vi "Run PPL Class Load Test.vi"(7 "Show UI on Class load?(T)":bool=TRUE, 8 "error in":errorcluster, 10 "PPL Class Test Plugins":refnum<class "PPL Class Test Plugin.lvclass">[](array[class]), 11 "PPL Name in PPL folder (entire PPL folder if empty)":string) -> (0 "error out":errorcluster, 1 "Success?":bool, 2 "Load Failure":string[](array[string]), 3 "Load Success":string[](array[string]))   [LabVIEW 2020, in "ProjectBuilder.lvlib"]
doc: "Get PPL paths and load the PPLs and see if load succeeds."
uses:
  ProjectBuilder.lvlib
  PPL/HDH.ClassLoader.lvlibp
  PPL Class Test Plugin/PPL Class Test Plugin.lvclass
panel:
  in  "Abort":bool
  out "Current class":string
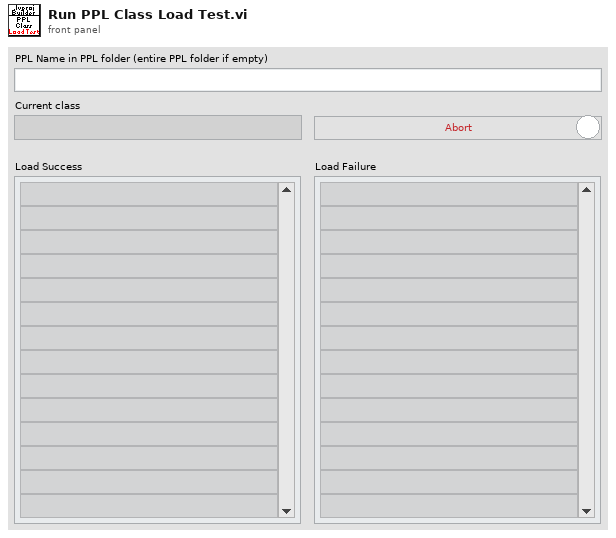
[diagram p1: front panel]
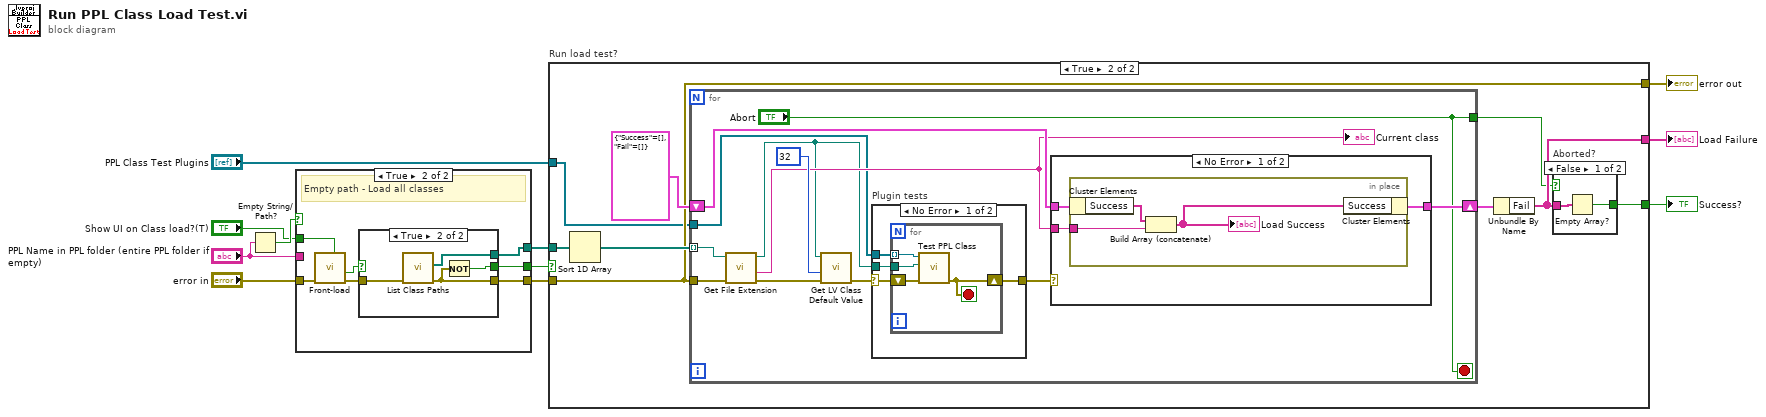
[diagram p0: block diagram]
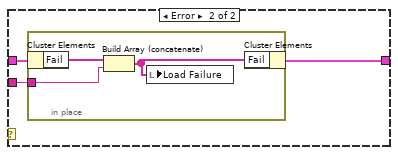
[diagram p5: hidden frame]
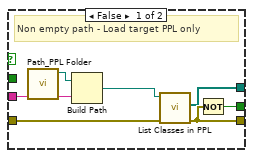
[diagram p6: hidden frame]
diagram:
  n1 = Empty String/Path?(string/path="PPL Name in PPL folder (entire PPL folder if empty)") -> (empty?=w11:bool)
  n2 = case shown="True" w11 {
    tunnel: [w17 w23] -> w8
    tunnel: "error in" -> [w18 w22]
    tunnel: [w16 w21] -> w6
    tunnel: [w15 w20] -> w7
    tunnel: "PPL Name in PPL folder (entire PPL folder if empty)" -> [w13 _]
    tunnel: "Show UI on Class load?(T)" -> [_ w19]
    frame False {
      # "Non empty path - Load target PPL only"
      n3 = call "Path_PPL Folder.vi"() -> ("Data Folder Path"=w14:path)  [unwired: 10 in, 1 out]
      n4 = Build Path(base path=w14, name or relative path=w13) -> (appended path=w12:path)
      n5 = call "List Classes in PPL.vi"("error in"=w18, "PPL Path"=w12) -> ("error out"=w16:errorcluster, "Class Path Array"=w15:path[])  [unwired: 7 in, 1 out]
      n6 = Not(x=w16) -> (.not. x?=w17:bool)
    }
    frame True {
      # "Empty path - Load all classes"
      n7 = call "Front-load.vi"("Show UI?(F)"=w19, "error in (no error)"=w22) -> ("error out"=w25:errorcluster, "Success?"=w24:bool)  [unwired: 8 in]
      n8 = case shown="True" w24 {
        selector: w24 -> [w27 _]
        tunnel: w25 -> [w26 w31]
        tunnel: [w27 w30] -> w23
        tunnel: [w26 w29] -> w21
        tunnel: [_ w28] -> w20
        frame False {
        }
        frame True {
          n9 = call "List Class Paths.vi"("error in (no error)"=w31) -> ("error out"=w29:errorcluster, "Class Paths"=w28:path[])  [unwired: 8 in, 1 out]
          n10 = Not(x=w29) -> (.not. x?=w30:bool)
        }
      }
    }
  }
  n11 = case "Run load test?" shown="True" w8 {
    selector: w8 -> [w33 _]
    tunnel: w7 -> [_ w42]
    tunnel: w6 -> [w32 w36]
    tunnel: [w33 w37] -> w4
    tunnel: [_ w38] -> w5
    tunnel: [w32 w36] -> w3
    tunnel: "PPL Class Test Plugins" -> [_ w34]
    frame False {
    }
    frame True {
      n12 = Sort 1D Array(array=w42) -> (sorted array=w41:path[])
      n13 = for {
        tunnel: w41 -> [w53] mode=indexing
        tunnel: w36 -> [w55]
        shift-right: [w50] -> w40
        shift-left: cluster{"Success":string[], "Fail":string[]} {"Success"=[], "Fail"=[]} -> [w52]
        tunnel: ["Abort"] -> w35
        tunnel: w34 -> [w48]
        stop <- "Abort" stop-if-true
        n14 = call <vilib>:"Get File Extension.vi"("error in (no error)"=w55, "file"=w53) -> ("error out"=w54:errorcluster, "filename without extension"=w51:string, "dup file"=w45:path)  [unwired: 5 in, 2 out]
        "Current class" <- w51
        n15 = call <vilib>:"Get LV Class Default Value.vi"("error in (no error)"=w54, "options"=u32 32, "class path"=w45) -> ("error out"=w47:errorcluster)  [unwired: 7 in, 1 out]
        n16 = case "Plugin tests" shown="No Error" w47 {
          selector: w47 -> [w59 w65]
          tunnel: w48 -> [w60 _]
          tunnel: [w58 w65] -> w46
          tunnel: w45 -> [w57 _]
          frame No Error {
            n17 = for {
              tunnel: w60 -> [w64] mode=indexing
              shift-right: [w61] -> w58
              shift-left: w59 -> [w62]
              tunnel: w57 -> [w63]
              stop <- w61 stop-if-true
              n18 = call-dynamic "Test PPL Class.vi"("error in (no error)"=w62, "File Path"=w63, "PPL Class Test Plugin in"=w64) -> ("error out"=w61:errorcluster)  [unwired: 8 in]
            }
          }
          frame Error {
          }
        }
        n19 = case shown="No Error" w46 {
          tunnel: w52 -> [w68 w74]
          tunnel: w51 -> [w67 w73]
          tunnel: [w66 w72] -> w50
          frame No Error {
            n20 = in-place {
              in-place-border: w67 -> [w70]
              n21 = in-place-cluster #1(w68) -> ("Success"=w71:string[])
              n22 = Build Array (concatenate)(w71, w70) -> (w69:string[])
              "Load Success" <- w69
              n23 = in-place-cluster #1("Success"=w69) -> (w66:cluster{"Success":string[], "Fail":string[]})
            }
          }
          frame Error {
            n24 = in-place {
              in-place-border: w73 -> [w76]
              n25 = in-place-cluster #2(w74) -> ("Fail"=w77:string[])
              n26 = Build Array (concatenate)(w77, w76) -> (w75:string[])
              n27 = local write "Load Failure"(w75) -> ()
              n28 = in-place-cluster #2("Fail"=w75) -> (w72:cluster{"Success":string[], "Fail":string[]})
            }
          }
        }
      }
      n29 = Unbundle By Name(w40) -> ("Fail"=w38:string[])
      n30 = case "Aborted?" shown="False" w35 {
        tunnel: w38 -> [w44 _]
        tunnel: [w43 _] -> w37
        frame False {
          n31 = Empty Array?(array=w44) -> (empty?=w43:bool)
        }
        frame True {
        }
      }
    }
  }
  "Load Failure" <- w5
  "Success?" <- w4
  "error out" <- w3
